vi "EnqueueMessage.vi"   [LabVIEW 2017, in "Server.lvlib" / "Message Queue.lvlib"]
doc: "For a regular message, enqueue the message. For a priority message, enqueue it at the front of the queue."
uses:
  Message Queue.lvlib
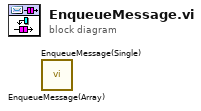
[diagram p0: block diagram]
diagram:
  n1 = call "EnqueueMessage(Array).vi"() -> ()  [unwired: 10 in, 2 out]
  n2 = call "EnqueueMessage(Single).vi"() -> ()  [unwired: 10 in, 2 out]
